vi "PTScanner.update DIM trendmsgs.vi"(0 "i ref in":refnum<vi>, 5 "error in":errorcluster) -> (14 "i ref out":refnum<vi>, 19 "error out":errorcluster)   [LabVIEW 2014, in "PTScanner.lvlib"]
uses:
  PTScanner.lvlib
  CSCore/BaseProcess/BaseProcess.event definition.ctl
  CSCore/CAEObj/CAEObj.event definition.ctl
  CSCore/BaseProcess/BaseProcess.descriptor string definition.ctl
  CSCore/BaseProcess/BaseProcess.lvlib
  CSCore/CAEObj/CAEObj.lvlib
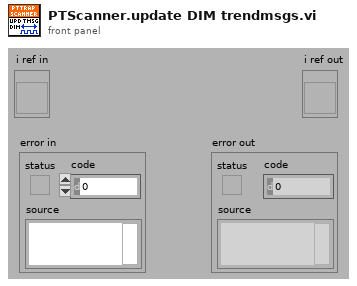
[diagram p1: front panel]
types:
  T1 = typedef "BaseProcess.lvlib/BaseProcess.event definition.ctl" = cluster{"CAEEvtDef":T2, "Data Descriptor":T3}
  T2 = typedef "CAEObj.lvlib/CAEObj.event definition.ctl" = cluster{"URL":string, "enable":bool, "ignoreResID":bool}
  T3 = typedef "BaseProcess.lvlib/BaseProcess.descriptor string definition.ctl" = string
  T4 = typedef "PTScanner.lvlib/PTScanner.i attribute.ctl" = cluster{"Object cmds":T5[], "Steps":cluster{"Finished":bool, "cmd setup":T6[]}[], "curStep":i32, "DIM IDs":cluster{"AllFinished":i32, "Finished":i32, "curStep":i32, "nofSteps":i32, "NomValues":i32[], "1D-Min":i32, "1D-Max":i32, "Dimensions":i32, "MaxDimensions":i32, "ScanedDeviceNames":i32[]}, "All Finished":bool, "DIMs in use":string[], "Running":bool, "Scan Delay":u32, "loop":bool, "Paused":bool, "Formed":bool}
  T5 = typedef "PTScanner.lvlib/PTScanner.obj parameters.ctl" = cluster{"object":string, "DIM address":string, "method":string, "data descriptor":string, "method parameters":cluster{"Name":string, "Descr":string, "Value":string, "Value?":bool}[], "Call Mode":enum16{"Simple DIM", "Synchronous"}, "actValue":dbl, "Centroid":dbl, "Minus Delta":dbl, "Plus Delta":dbl, "increment":dbl, "DIM Status":cluster{"no link":bool, "quality":i32, "Time Stamp":timestamp}, "range":dbl, "DIMChannelIndex":i32}
  T6 = typedef "PTScanner.lvlib/PTScanner.step obj parameters.ctl" = cluster{"obj index":i32, "nomValue":dbl, "fulfilled":bool}
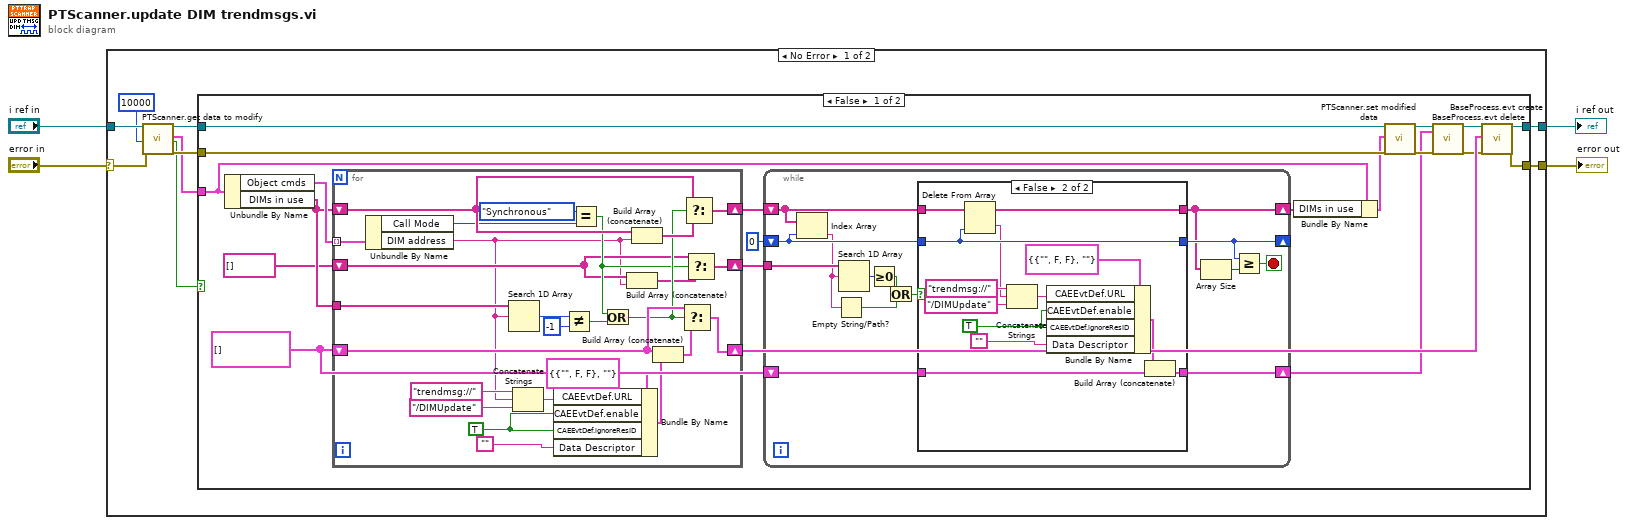
[diagram p0: block diagram]
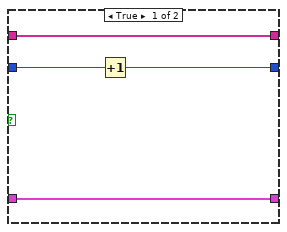
[diagram p2: hidden frame]
diagram:
  n1 = case shown="No Error" "error in" {
    selector: "error in" -> [w11 w93]
    tunnel: "i ref in" -> [w7 w94]
    tunnel: [w13 w94] -> w3
    tunnel: [w12 w93] -> w2
    frame No Error {
      n2 = call "PTScanner.get data to modify.vi"("i ref in"=w7, "ms timeout (10000)"=10000, "error in (no error)"=w11) -> ("i ref out"=w8:refnum<vi>, "i attribute"=w9:T4, "timed out"=w5:bool, "error out"=w10:errorcluster)  [unwired: 13 in]
      n3 = case shown="False" w5 {
        tunnel: [w33 w91] -> w13
        tunnel: [w32 w92] -> w12
        tunnel: w10 -> [w28 w92]
        tunnel: w9 -> [w27 _]
        tunnel: w8 -> [w29 w91]
        frame False {
          w18 = T1[] []
          n4 = Unbundle By Name(w27) -> ("Object cmds"=w30:T5[], "DIMs in use"=w26:string[])
          n5 = for {
            tunnel: w30 -> [w83] mode=indexing
            shift-right: [w77] -> w31
            shift-left: w18 -> [w79]
            tunnel: w26 -> [w82]
            shift-right: [w76] -> w24
            shift-left: w26 -> [w75]
            shift-right: [w70] -> w14
            shift-left: string[] [] -> [w67]
            w89 = TRUE ("CAEEvtDef.ignoreResID")
            n6 = Unbundle By Name(w83) -> ("Call Mode"=w72:enum16{"Simple DIM", "Synchronous"}, "DIM address"=w66:string)
            n7 = Search 1D Array(1D array=w82, element=w66) -> (index of element=w81:i32)  [unwired: 1 in]
            n8 = Concatenate Strings("trendmsg://", w66, "/DIMUpdate" ("string")) -> (w86:string)
            n9 = Bundle By Name(cluster=T1 {"CAEEvtDef"={"URL"="", "enable"=FALSE, "ignoreResID"=FALSE}, "Data Descriptor"=""} ("event definition"), "CAEEvtDef.URL"=w86, "CAEEvtDef.enable"=w89, "CAEEvtDef.ignoreResID"=w89, "Data Descriptor"="") -> (w84:T1)
            n10 = Not Equal?(x=w81, y=-1) -> (x != y?=w73:bool)
            n11 = Equal?(x=enum16{"Simple DIM", "Synchronous"}."Synchronous" ("Call Mode"), y=w72) -> (x = y?=w68:bool)
            n12 = Or(x=w68, y=w73) -> (x .or. y?=w69:bool)
            n13 = Build Array (concatenate)(w67, w66) -> (w65:string[])
            n14 = Build Array (concatenate)(w75, w66) -> (w74:string[])
            n15 = Build Array (concatenate)(w79, w84) -> (w78:T1[])
            n16 = Select(t=w79, s=w69, f=w78) -> (s? t:f=w77:T1[])
            n17 = Select(t=w75, s=w69, f=w74) -> (s? t:f=w76:string[])
            n18 = Select(t=w67, s=w68, f=w65) -> (s? t:f=w70:string[])
          }
          n19 = while {
            tunnel: w14 -> [w47]
            shift-right: [w40] -> w16
            shift-left: w24 -> [w46]
            shift-right: [w41] -> _
            shift-left: 0 -> [w45]
            shift-right: [w43] -> w17
            shift-left: w18 -> [w44]
            stop <- w39 stop-if-true
            n20 = Index Array(array=w46, index=w45) -> (element=w38:string)
            n21 = Empty String/Path?(string/path=w38) -> (empty?=w36:bool)
            n22 = Search 1D Array(1D array=w47, element=w38) -> (index of element=w37:i32)  [unwired: 1 in]
            n23 = Greater Or Equal To 0?(x=w37) -> (x >= 0?=w35:bool)
            n24 = Or(x=w35, y=w36) -> (x .or. y?=w34:bool)
            n25 = case shown="False" w34 {
              tunnel: w46 -> [w51 w64]
              tunnel: [w51 w63] -> w40
              tunnel: w45 -> [w50 w62]
              tunnel: [w49 w62] -> w41
              tunnel: w44 -> [w48 w55]
              tunnel: [w48 w54] -> w43
              frame True {
                n26 = Increment(x=w50) -> (x+1=w49:i32)
              }
              frame False {
                w57 = TRUE ("CAEEvtDef.ignoreResID")
                n27 = Delete From Array(array=w64, index=w62) -> (deleted portion=w52:string, array with subset deleted=w63:string[])  [unwired: 1 in]
                n28 = Concatenate Strings("trendmsg://", w52, "/DIMUpdate" ("string")) -> (w58:string)
                n29 = Bundle By Name(cluster=T1 {"CAEEvtDef"={"URL"="", "enable"=FALSE, "ignoreResID"=FALSE}, "Data Descriptor"=""} ("event definition"), "CAEEvtDef.URL"=w58, "CAEEvtDef.enable"=w57, "CAEEvtDef.ignoreResID"=w57, "Data Descriptor"="") -> (w53:T1)
                n30 = Build Array (concatenate)(w53, w55) -> (w54:T1[])
              }
            }
            n31 = Array Size(array=w40) -> (size(s)=w42:i32)
            n32 = Greater Or Equal?(x=w41, y=w42) -> (x >= y?=w39:bool)
          }
          n33 = Bundle By Name(cluster=w27, "DIMs in use"=w16) -> (w25:T4)
          n34 = call "PTScanner.set modified data.vi"("i ref in"=w29, "CLASS.i attribute"=w25, "error in (no error)"=w28) -> ("i ref out"=w22:refnum<vi>, "error out"=w20:errorcluster)  [unwired: 15 in]
          n35 = call "BaseProcess.evt delete.vi"("i ref in"=w22, "events"=w17, "error in (no error)"=w20) -> ("i ref out"=w21:refnum<vi>, "error out"=w19:errorcluster)  [unwired: 13 in, 2 out]
          n36 = call "BaseProcess.evt create.vi"("i ref in"=w21, "newEvents"=w31, "error in (no error)"=w19) -> ("i ref out"=w33:refnum<vi>, "error out"=w32:errorcluster)  [unwired: 13 in, 2 out]
        }
        frame True {
        }
      }
    }
    frame Error {
    }
  }
  "i ref out" <- w3
  "error out" <- w2
